vi "BRig_dataExp_T_Reward_min_R.vi"() -> (2 "output_T_Reward_min_R":i32)   [LabVIEW 2014]
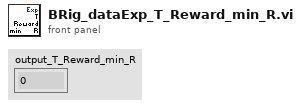
[diagram p1: front panel]
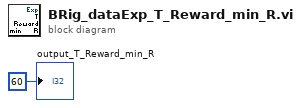
[diagram p0: block diagram]
diagram:
  "output_T_Reward_min_R" <- 60 ("output_iBlock")
